vi "PIByteFiles.vi"(0 "use min z value?":bool, 4 "Final Sector Image Size":T1={"x"=346, "y"=240, "Trim image sides?"=TRUE, "start trim"=45, "end trim line"=256}, 5 "Scan Info":T4 {"delay" format="%.2f"; "pivot distance" format="%.2f"; "sector scan angle" format="%.2f"}, 6 "Pre scale?":bool=TRUE, 7 "Smooth factor":i32=3, 8 "Data Type":u16(ring) items=["midband", "slope", "intercept"], 9 "Range Params":T2={"mb max"=-10.0, "mb min"=-60.0, "slope max"=4.0, "slope min"=-8.0, "int max"=5.0, "int min"=-85.0} {"int min" format="%.2f"; "int max" format="%.2f"; "slope min" format="%.2f"; "slope max" format="%.2f"; "mb min" format="%.2f"; "mb max" format="%.2f"}, 10 "A/D info":T3, 11 "raw image data in":dbl[][](array[numeric]) format="%.2f") -> (2 "Scaled Image Data":u8[][](array[numeric]), 3 "raw sector out":dbl[][](array[numeric]))   [LabVIEW 2022 SP3]
uses:
  <vilib>/Analysis/NI_AALPro.lvlib
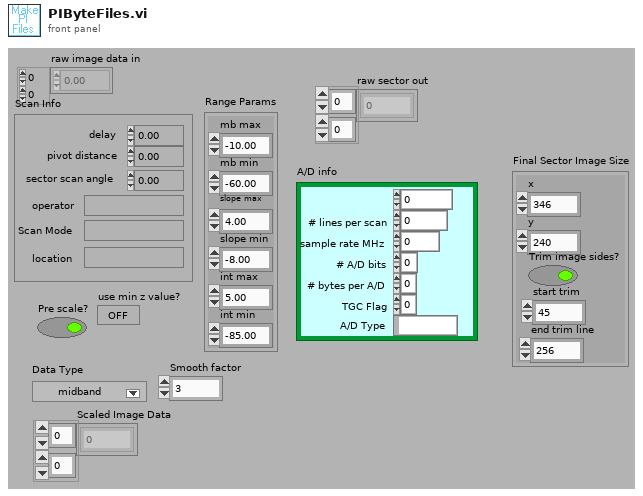
[diagram p1: front panel]
types:
  T1 = cluster{"x":i32, "y":i32, "Trim image sides?":bool, "start trim":i32, "end trim line":i32}
  T2 = cluster{"mb max":dbl, "mb min":dbl, "slope max":dbl, "slope min":dbl, "int max":dbl, "int min":dbl}
  T3 = cluster{"# rf points per line":u16, "# lines per scan":u16, "sample rate MHz":u16, "# A/D bits":i16, "# bytes per A/D":u16, "TGC Flag":u16, "A/D Type":string}
  T4 = cluster{"delay":sgl, "pivot distance":sgl, "sector scan angle":sgl, "operator":string, "Scan Mode":string, "location":string}
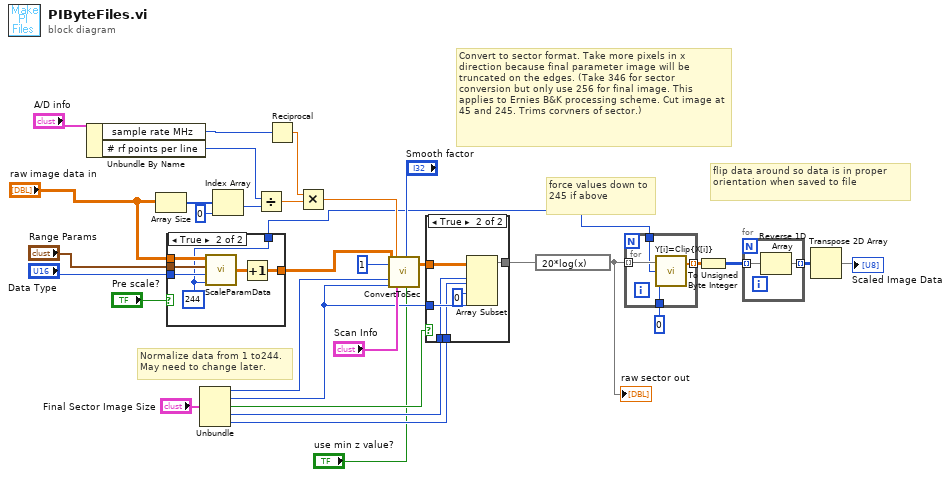
[diagram p0: block diagram]
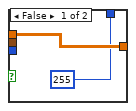
[diagram p2: hidden frame]
diagram:
  # "force values down to 245 if above"
  # "flip data around so data is in proper orientation when saved to file"
  # "Convert to sector format. Take more pixels in x direction because final parameter image will be truncated on the edges. (Take 346 for sector conversion but only use 256 for final image. This applies to Ernies B&K processing scheme. Cut image at 45 and 245. Trims corvners of sector.)"
  # "Normalize data from 1 to244.\nMay need to change later."
  n1 = Unbundle By Name("A/D info") -> ("sample rate MHz"=w26:u16, "# rf points per line"=w27:u16)
  n2 = Array Size(array="raw image data in") -> (size(s)=w32:i32[])
  n3 = case shown="True" "Pre scale?" {
    tunnel: "Data Type" -> [_ w41]
    tunnel: "Range Params" -> [_ w40]
    tunnel: [w35 w36] -> w2
    tunnel: "raw image data in" -> [w35 w39]
    tunnel: [255 w38] -> w7
    frame False {
    }
    frame True {
      w38 = 244
      n4 = call "ScaleParamData.vi"("max scale value"=w38, "parameter"=w41, "Range Params"=w40, "raw image data in"=w39) -> ("scaled output"=w37:dbl[][])
      n5 = Increment(x=w37) -> (x+1=w36:dbl[][])
    }
  }
  n6 = Unbundle("Final Sector Image Size") -> ("x"=w15:i32, "y"=w14:i32, "Trim image sides?"=w13:bool, "start trim"=w12:i32, "end trim line"=w11:i32)
  n7 = Index Array(array=w32, index=0 ("Index")) -> (element=w33:i32)
  n8 = Divide(x=w27, y=w33) -> (x/y=w25:dbl)
  n9 = Reciprocal(x=w26) -> (1/x=w24:dbl)
  n10 = Multiply(x=w24, y=w25) -> (x*y=w30:dbl)
  n11 = call "ConvertToSec.vi"("raw image data in"=w2, "reduce pts by factor of"=1, "pixels in x"=w15, "pixels in y"=w14, "Time between rf pts\nmicros"=w30, "Scan Info"="Scan Info", "Smooth factor"="Smooth factor", "use min z value?"="use min z value?") -> ("raw sector out"=w3:dbl[][])  [unwired: 3 in, 8 out]
  n12 = case shown="True" w13 {
    tunnel: [w42 w48] -> w6
    tunnel: w3 -> [w42 w46]
    tunnel: w14 -> [_ w45]
    tunnel: w12 -> [_ w44]
    tunnel: w11 -> [_ w43]
    frame False {
    }
    frame True {
      n13 = Array Subset(array=w46, index (row)=w44, length (row)=w43, index (col)=0 ("Array Index"), length (col)=w45) -> (w48:dbl[][])
    }
  }
  n14 = expression code="20*log(x)"(w6) -> (w1:dbl[][])
  "raw sector out" <- w1
  n15 = for {
    tunnel: w1 -> [w52] mode=indexing
    tunnel: [w51] -> w21 mode=indexing
    tunnel: w7 -> [w50]
    tunnel: 0 -> [w49]
    n16 = call <vilib>:"Y[i]=Clip{X[i]}.vi"("lower limit"=w49, "upper limit"=w50, "Input Array"=w52) -> ("Clipped Array"=w51:dbl[])  [unwired: 1 out]
  }
  n17 = To Unsigned Byte Integer(number=w21) -> (unsigned 8bit integer=w17:u8[][])
  n18 = for {
    tunnel: w17 -> [w54] mode=indexing
    tunnel: [w53] -> w22 mode=indexing
    n19 = Reverse 1D Array(array=w54) -> (reversed array=w53:u8[])
  }
  n20 = Transpose 2D Array(2D array=w22) -> (transposed array=→"Scaled Image Data":u8[][])
